vi "feed_back.vi"() -> ()   [LabVIEW 2017]
panel:
  in  "PWM":dbl
  out "光强":dbl
  out "c":dbl
  out "b":dbl
  out "a":dbl
  in  "传感器编号":i32
  in  "灯板编号":i32
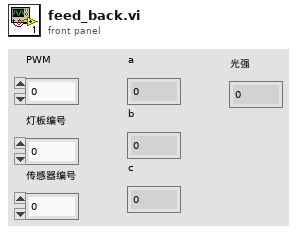
[diagram p1: front panel]
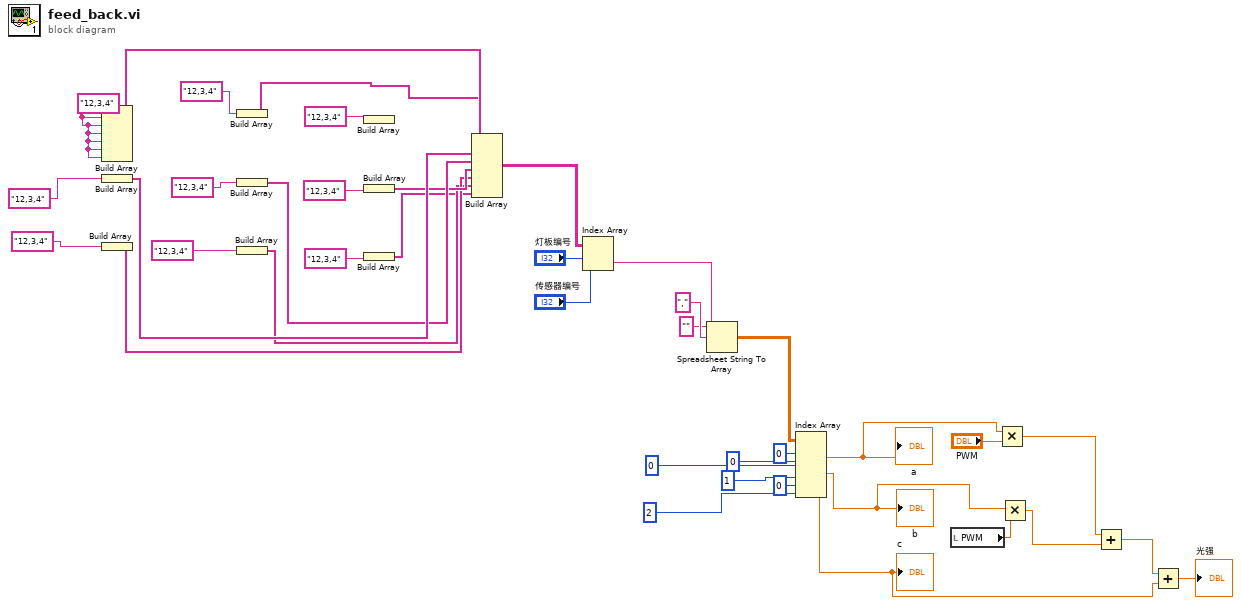
[diagram p0: block diagram]
diagram:
  w39 = "12,3,4"
  n1 = Build Array(w39, w39, w39, w39, w39, w39, w39) -> (w38:string[])
  n2 = Build Array("12,3,4") -> (w27:string[])
  n3 = Build Array("12,3,4") -> (w24:string[])
  n4 = Build Array("12,3,4") -> (w28:string[])
  n5 = Build Array("12,3,4") -> (w26:string[])
  n6 = Build Array("12,3,4") -> (w23:string[])
  n7 = Build Array("12,3,4") -> ()  [unwired: 1 out]
  n8 = Build Array("12,3,4") -> (w25:string[])
  n9 = Build Array("12,3,4") -> (w22:string[])
  n10 = Build Array(w38, w28, w27, w26, w25, w24, w23, w22) -> (w37:string[][])
  n11 = Index Array(array=w37, index (row)="灯板编号", index (col)="传感器编号") -> (element=w19:string)
  n12 = Spreadsheet String To Array(delimiter (Tab)="," ("分隔符(Tab)"), format string="" ("格式字符串"), spreadsheet string=w19) -> (array=w16:dbl[][])  [unwired: 1 in]
  n13 = Index Array(array=w16, index (row) #1=0 ("索引 (行)"), index (col) #1=0 ("禁用的索引 (列)"), index (row) #2=0 ("索引 (行)"), index (col) #2=1 ("禁用的索引 (列)"), index (row) #3=0 ("禁用的索引 (行)"), index (col) #3=2 ("索引 (列)")) -> (element #1=w9:dbl, element #2=w8:dbl, element #3=w4:dbl)
  "a" <- w9
  "b" <- w8
  "c" <- w4
  n14 = local read "PWM"() -> (w1:dbl)
  n15 = Multiply(x=w9, y="PWM") -> (x*y=w7:dbl)
  n16 = Multiply(x=w8, y=w1) -> (x*y=w6:dbl)
  n17 = Add(x=w7, y=w6) -> (x+y=w5:dbl)
  n18 = Add(x=w5, y=w4) -> (x+y=→"光强":dbl)
